vi "AmplifierTest.vi"() -> ()   [LabVIEW 2020]
panel:
  out "Output Subunits":u32
  out "Input Subunits":u32
  in  "Gain (x1)":u32(ring)=1 items=["x1"=1, "x2"=2, "x5"=3, "x7"=4, "x10"=5, "x14"=6, "x20"=7]
  in  "Channel (CH1)":u32(ring)=1 items=["CH1"=1, "CH2"=2, "CH3"=3, "CH4"=4, "CH5"=5]
  out "self-test message":string
  in  "resource name":refnum<visa-resource-name>="PXI23::10::INSTR"
  out "self test result":i16 format="%.0g"
  out "ID String":string
  out "error out":errorcluster
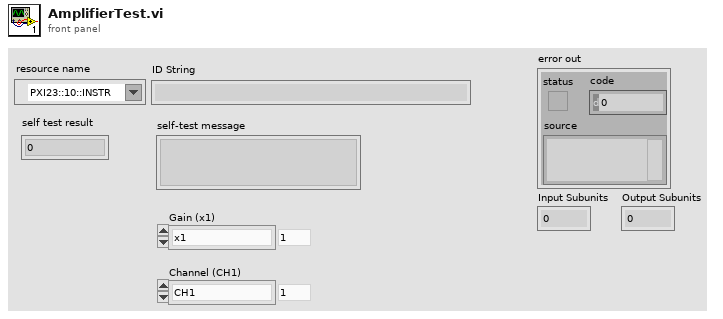
[diagram p1: front panel]
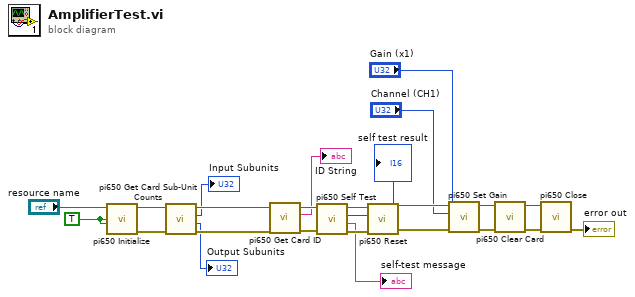
[diagram p0: block diagram]
diagram:
  w16 = TRUE ("id query (Do Query)")
  n1 = call <instrlib>:"pi650 Initialize.vi"("reset device (Reset Device)"=w16, "id query (Do Query)"=w16, "resource name"="resource name") -> ("error out"=w6:errorcluster, "instrument handle out"=w5:refnum<visa-resource-name>)  [unwired: 7 in]
  n2 = call <instrlib>:"pi650 Get Card Sub-Unit Counts.vi"("error in (no error)"=w6, "instrument handle"=w5) -> ("error out"=w4:errorcluster, "Output Subunits"=→"Output Subunits":u32, "Input Subunits"=→"Input Subunits":u32, "instrument handle out"=w3:refnum<visa-resource-name>)  [unwired: 6 in]
  n3 = call <instrlib>:"pi650 Get Card ID.vi"("error in (no error)"=w4, "instrument handle"=w3) -> ("error out"=w23:errorcluster, "ID String"=→"ID String":string, "instrument handle out"=w24:refnum<visa-resource-name>)  [unwired: 7 in]
  n4 = call <instrlib>:"pi650 Self Test.vi"("error in (no error)"=w23, "instrument handle"=w24) -> ("error out"=w22:errorcluster, "self-test message"=→"self-test message":string, "self test result"=→"self test result":i16, "instrument handle out"=w21:refnum<visa-resource-name>)  [unwired: 6 in]
  n5 = call <instrlib>:"pi650 Reset.vi"("error in (no error)"=w22, "instrument handle"=w21) -> ("error out"=w9:errorcluster, "instrument handle out"=w10:refnum<visa-resource-name>)  [unwired: 8 in]
  n6 = call <instrlib>:"pi650 Set Gain.vi"("error in (no error)"=w9, "Gain (x1)"="Gain (x1)", "Channel (CH1)"="Channel (CH1)", "instrument handle"=w10) -> ("error out"=w12:errorcluster, "instrument handle out"=w11:refnum<visa-resource-name>)  [unwired: 6 in]
  n7 = call <instrlib>:"pi650 Clear Card.vi"("error in (no error)"=w12, "instrument handle"=w11) -> ("error out"=w14:errorcluster, "instrument handle out"=w13:refnum<visa-resource-name>)  [unwired: 8 in]
  n8 = call <instrlib>:"pi650 Close.vi"("error in (no error)"=w14, "instrument handle"=w13) -> ("error out"=→"error out":errorcluster)  [unwired: 9 in]
